vi "HexToHexString.vi"(7 "Way":bool, 10 "Data":string) -> (2 "String":string)   [LabVIEW 2013]
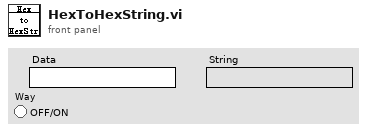
[diagram p1: front panel]
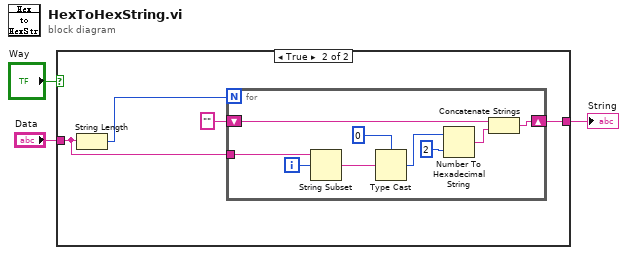
[diagram p0: block diagram]
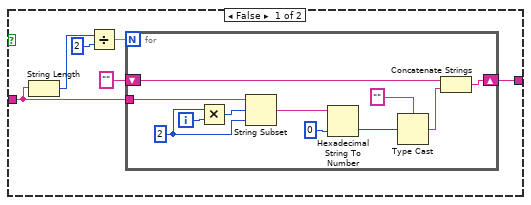
[diagram p2: hidden frame]
diagram:
  n1 = case shown="True" "Way" {
    tunnel: "Data" -> [w5 w24]
    tunnel: [w4 w21] -> w2
    frame False {
      n2 = String Length(string=w5) -> (length=w7:i32)
      n3 = Divide(x=w7, y=2) -> (x/y=w9:dbl)
      n4 = for {
        N: w9 -> [_]
        tunnel: w5 -> [w14]
        shift-right: [w15] -> w4
        shift-left: "" -> [w17]
        i -> [w13]
        w12 = 2 ("length (rest)")
        n5 = Multiply(x=w12, y=w13) -> (x*y=w11:i32)
        n6 = String Subset(string=w14, offset (0)=w11, length (rest)=w12) -> (substring=w10:string)
        n7 = Hexadecimal String To Number(string=w10, default (0uL)=u8 0 ("default (0 U32)")) -> (number=w18:u8)  [unwired: 2 out]
        n8 = Type Cast(type="", x=w18) -> (*(type *) &x=w16:string)
        n9 = Concatenate Strings(w17, w16) -> (w15:string)
      }
    }
    frame True {
      n10 = String Length(string=w24) -> (length=w22:i32)
      n11 = for {
        N: w22 -> [_]
        tunnel: w24 -> [w31]
        shift-right: [w26] -> w21
        shift-left: "" -> [w28]
        i -> [w29]
        n12 = String Subset(string=w31, offset (0)=w29) -> (substring=w30:string)  [unwired: 1 in]
        n13 = Type Cast(type=u8 0 ("default (0 U32)"), x=w30) -> (*(type *) &x=w32:u8)
        n14 = Number To Hexadecimal String(1:i16 2 ("width (-)"), 2:w32) -> (0:w27:string)
        n15 = Concatenate Strings(w28, w27) -> (w26:string)
      }
    }
  }
  "String" <- w2
